vi "Get Panel Image and Origin.vi"(8 "error in (no error)":errorcluster, 10 "Bit Depth":enum16{"1-bit", "4-bit", "8-bit", "24-bit"}(ring)=enum."24-bit", 11 "vi name":string) -> (0 "error out":errorcluster, 1 "FP.Origin":cluster{"Horizontal":i16, "Vertical":i16}, 2 "FP.Bounds":T2, 3 "image data":T1)   [LabVIEW 2011]
uses:
  <vilib>/picture/picture.llb/imagedata.ctl
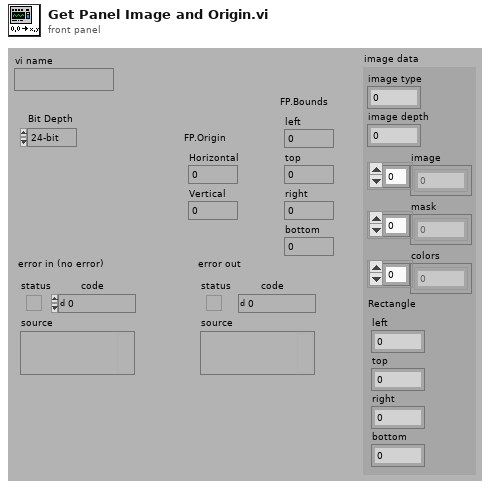
[diagram p1: front panel]
types:
  T1 = typedef "imagedata.ctl" = cluster{"image type":i32, "image depth":i32, "image":u8[], "mask":u8[], "colors":u32[], "Rectangle":cluster{"left":i16, "top":i16, "right":i16, "bottom":i16}}
  T2 = cluster{"left":i16, "top":i16, "right":i16, "bottom":i16}
  T3 = typedef "LVPointTypeDef.ctl" = cluster{"Horizontal":i16, "Vertical":i16}
  T4 = typedef "LVRectTypeDef.ctl" = cluster{"left":i16, "top":i16, "right":i16, "bottom":i16}
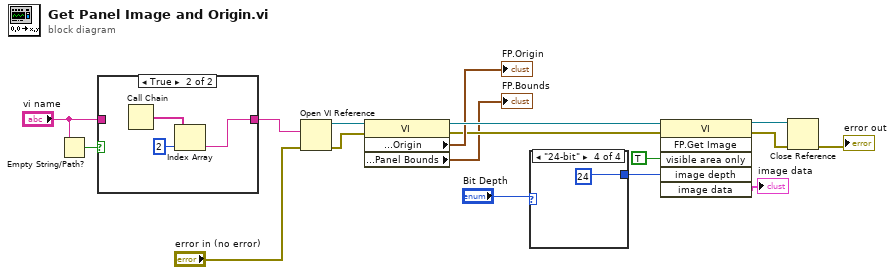
[diagram p0: block diagram]
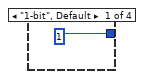
[diagram p3: hidden frame]
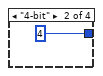
[diagram p4: hidden frame]
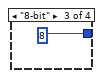
[diagram p5: hidden frame]
diagram:
  n1 = Empty String/Path?(string/path="vi name") -> (empty?=w6:bool)
  n2 = case shown="True" w6 {
    tunnel: [w18 w19] -> w4
    tunnel: "vi name" -> [w18 _]
    frame False {
    }
    frame True {
      n3 = Call Chain() -> (call chain=w21:string[])
      n4 = Index Array(array=w21, index=2) -> (element=w19:string)
    }
  }
  n5 = Open VI Reference(vi path=w4, error in (no error)="error in (no error)") -> (vi reference=w11:refnum<vi>, error out=w7:errorcluster)  [unwired: 4 out]
  n6 = property class="VI"(reference=w11, error in=w7) -> (reference out=w10:refnum<vi>, error out=w8:errorcluster, "Front Panel Window:Origin"=→"FP.Origin":T3, "Front Panel Window:Panel Bounds"=→"FP.Bounds":T4)
  n7 = case shown="\"24-bit\"" "Bit Depth" {
    tunnel: [1 4 8 24] -> w17
    frame "1-bit", Default {
    }
    frame "4-bit" {
    }
    frame "8-bit" {
    }
    frame "24-bit" {
    }
  }
  n8 = invoke class="VI" method="FP.Get Image"(reference=w10, error in=w8, "visible area only"=TRUE, "image depth"=w17) -> (reference out=w16:refnum<vi>, error out=w15:errorcluster, "image data"=→"image data":T1)  [unwired: 2 in, 3 out]
  n9 = Close Reference(reference=w16, error in (no error)=w15) -> (error out=→"error out":errorcluster)
